vi "Parse Headers.vi"(5 "Headers":string, 11 "error in (no error)":errorcluster) -> (6 "Parsed headers":variant, 15 "error out":errorcluster)   [LabVIEW 2023, in "Weather Request Loop.lvlib"]
doc: "Parses the header block from an HTTP response without the response code. Returns a variant containing the parsed headers. The variant contains an attribute for each header, with the name of each attribute corresponding to the name of a header, converted to lower case. The value of each attribute is the value of that corresponding header."
uses:
  Weather Request Loop.lvlib
  <vilib>/Utility/error.llb/Trim Whitespace One-Sided.vi
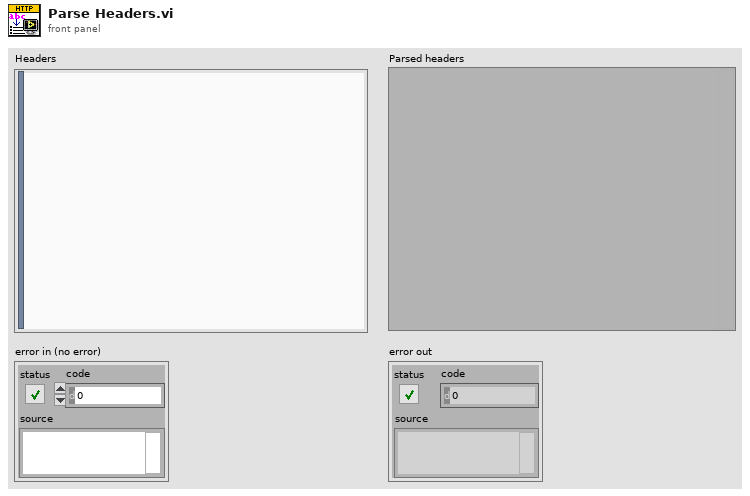
[diagram p1: front panel]
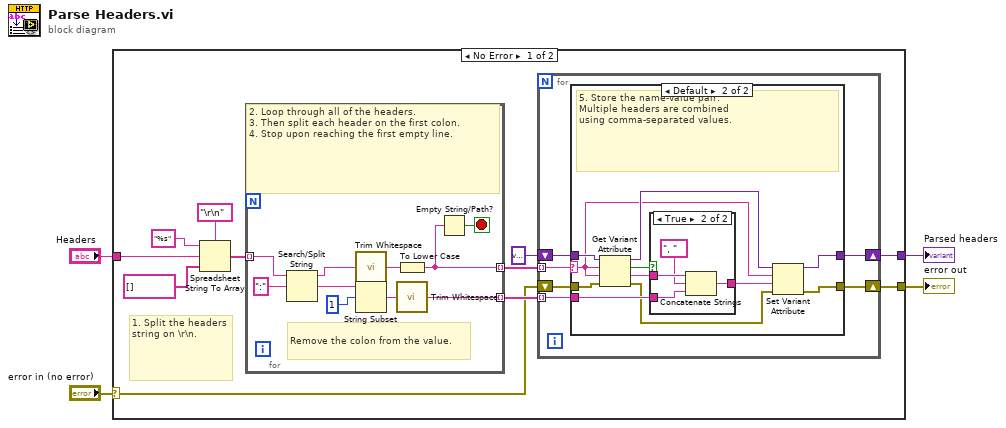
[diagram p0: block diagram]
diagram:
  n1 = case shown="No Error" "error in (no error)" {
    selector: "error in (no error)" -> [w7 w50]
    tunnel: [w6 w50] -> w4
    tunnel: "Headers" -> [w11 _]
    tunnel: [w5 _] -> w2
    frame No Error {
      # "1. Split the headers string on \\r\\n."
      n2 = Spreadsheet String To Array(delimiter (Tab)="\r\n", format string="%s", spreadsheet string=w11, array type (2D Dbl)=string[] []) -> (array=w15:string[])
      n3 = for {
        tunnel: w15 -> [w43] mode=indexing
        tunnel: [w40] -> w10 mode=indexing
        tunnel: [w45] -> w9 mode=indexing
        stop <- w41 stop-if-true
        # "Remove the colon from the value."
        # "2. Loop through all of the headers.\n3. Then split each header on the first colon.\n4. Stop upon reaching the first empty line."
        n4 = Search/Split String(string=w43, search string/char (-)=":") -> (substring before match=w42:string, match + rest of string=w48:string)  [unwired: 1 in, 1 out]
        n5 = call <vilib>:"Trim Whitespace.vi"("string"=w42) -> ("trimmed string"=w46:string)  [unwired: 1 in]
        n6 = String Subset(string=w48, offset (0)=1) -> (substring=w44:string)  [unwired: 1 in]
        n7 = To Lower Case(string=w46) -> (all lower case string=w40:string)
        n8 = call <vilib>:"Trim Whitespace.vi"("string"=w44) -> ("trimmed string"=w45:string)  [unwired: 1 in]
        n9 = Empty String/Path?(string/path=w40) -> (empty?=w41:bool)
      }
      n10 = for {
        tunnel: w10 -> [w21] mode=indexing
        tunnel: w9 -> [w19] mode=indexing
        shift-right: [w16] -> w5
        shift-left: variant ("Parsed headers") -> [w20]
        shift-right: [w17] -> w6
        shift-left: w7 -> [w18]
        n11 = case shown="Default" w21 {
          selector: w21 -> [_ w24]
          tunnel: [w22 w29] -> w16
          tunnel: w19 -> [_ w30]
          tunnel: w18 -> [w23 w31]
          tunnel: [w23 w28] -> w17
          tunnel: w20 -> [w22 w34]
          frame "" {
            # "Ignore empty lines."
          }
          frame Default {
            # "5. Store the name-value pair.\nMultiple headers are combined\nusing comma-separated values."
            n12 = Get Variant Attribute(Variant=w34, name=w24, default value (empty Variant)=w24, error in=w31) -> (duplicate Variant=w27:variant, found=w33:bool, value=w32:string, error out=w25:errorcluster)
            n13 = case shown="True" w33 {
              tunnel: w32 -> [_ w39]
              tunnel: w30 -> [w35 w38]
              tunnel: [w35 w36] -> w26
              frame False {
              }
              frame True {
                n14 = Concatenate Strings(w39, ", " ("string"), w38) -> (w36:string)
              }
            }
            n15 = Set Variant Attribute(Variant=w27, name=w24, value=w26, error in=w25) -> (Variant out=w29:variant, error out=w28:errorcluster)  [unwired: 1 out]
          }
        }
      }
    }
    frame Error {
    }
  }
  "error out" <- w4
  "Parsed headers" <- w2
